vi "Profile Auton - Distance.vi"(8 "error in (no error)":errorcluster, 10 "Time (s)":dbl format="%#_13g", 11 "Distance (ft)":dbl) -> (0 "error out":errorcluster)   [LabVIEW 2017]
uses:
  Robot Global Data.vi
  <vilib>/Rock Robotics/WPI/Utilities/WPI_GetSetVariantRefNum.vi
  <vilib>/Rock Robotics/Network Tables/NT Write Number.vi
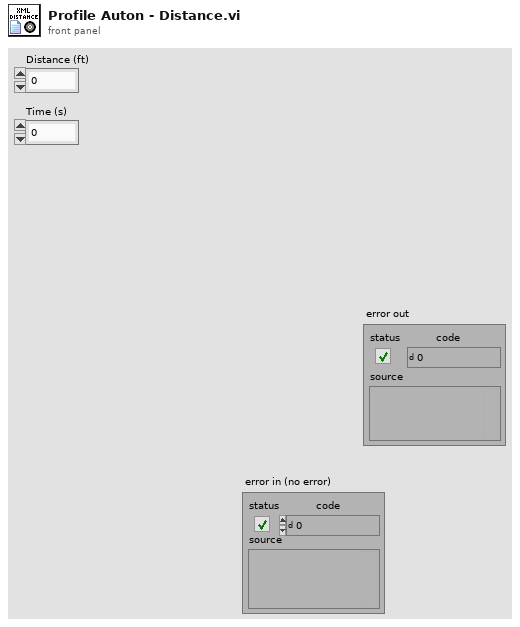
[diagram p1: front panel]
types:
  T1 = typedef "WPI_MotorControlDeviceRef.ctl" = cluster{"DeviceStatus":errorcluster, "Type":T2, "PWM":cluster{"PWM Channel":T3, "DeadBand":T4}, "CAN":cluster{"Device Number":u8, "SetOutput VI Ref":variant, "GetOutput VI Ref":variant, "Enable VI Ref":variant, "Disable VI Ref":variant, "Data":variant}, "Invert":bool, "DIO PWM":cluster{"PWM \"Enable\" Channel":T3, "DIOChannel":T5, "PWM Rate":dbl}}
  T2 = typedef "WPI_MotorControlType.ctl" = enum16{"PWM", "CAN", "DIO PWM"}
  T3 = typedef "FPGA_DIOPWMChannel.ctl" = enum8{"PWM 0", "PWM 1", "PWM 2", "PWM 3", "PWM 4", "PWM 5", "PWM 6", "PWM 7", "PWM 8", "PWM 9", "PWM MXP 0", "PWM MXP 1", "PWM MXP 2", "PWM MXP 3", "PWM MXP 4", "PWM MXP 5", "PWM MXP 6", "PWM MXP 7", "PWM MXP 8", "PWM MXP 9", "Invalid"}
  T4 = typedef "WPI_PWMDeadband.ctl" = cluster{"Name":string, "maxPositivePwm":i32, "minPositivePwm":i32, "centerPwm":i32, "maxNegativePwm":i32, "minNegativePwm":i32, "angularRange":u16}
  T5 = typedef "FPGA_DIOChannel.ctl" = enum8{"DIO 0", "DIO 1", "DIO 2", "DIO 3", "DIO 4", "DIO 5", "DIO 6", "DIO 7", "DIO 8", "DIO 9", "DIO MXP 0", "DIO MXP 1", "DIO MXP 2", "DIO MXP 3", "DIO MXP 4", "DIO MXP 5", "DIO MXP 6", "DIO MXP 7", "DIO MXP 8", "DIO MXP 9", "DIO MXP 10", "DIO MXP 11", "DIO MXP 12", "DIO MXP 13", "DIO MXP 14", "DIO MXP 15", "SPI Port CS1", "SPI Port CS2", "SPI Port CS3", "SPI Port MISO", "SPI Port MOSI", "Invalid"}
  T6 = typedef "WPI_RobotDriveDevRef.ctl" = cluster{"DevStatus":errorcluster, "Motors[]":T1[], "Square Inputs":bool, "Max Output":dbl}
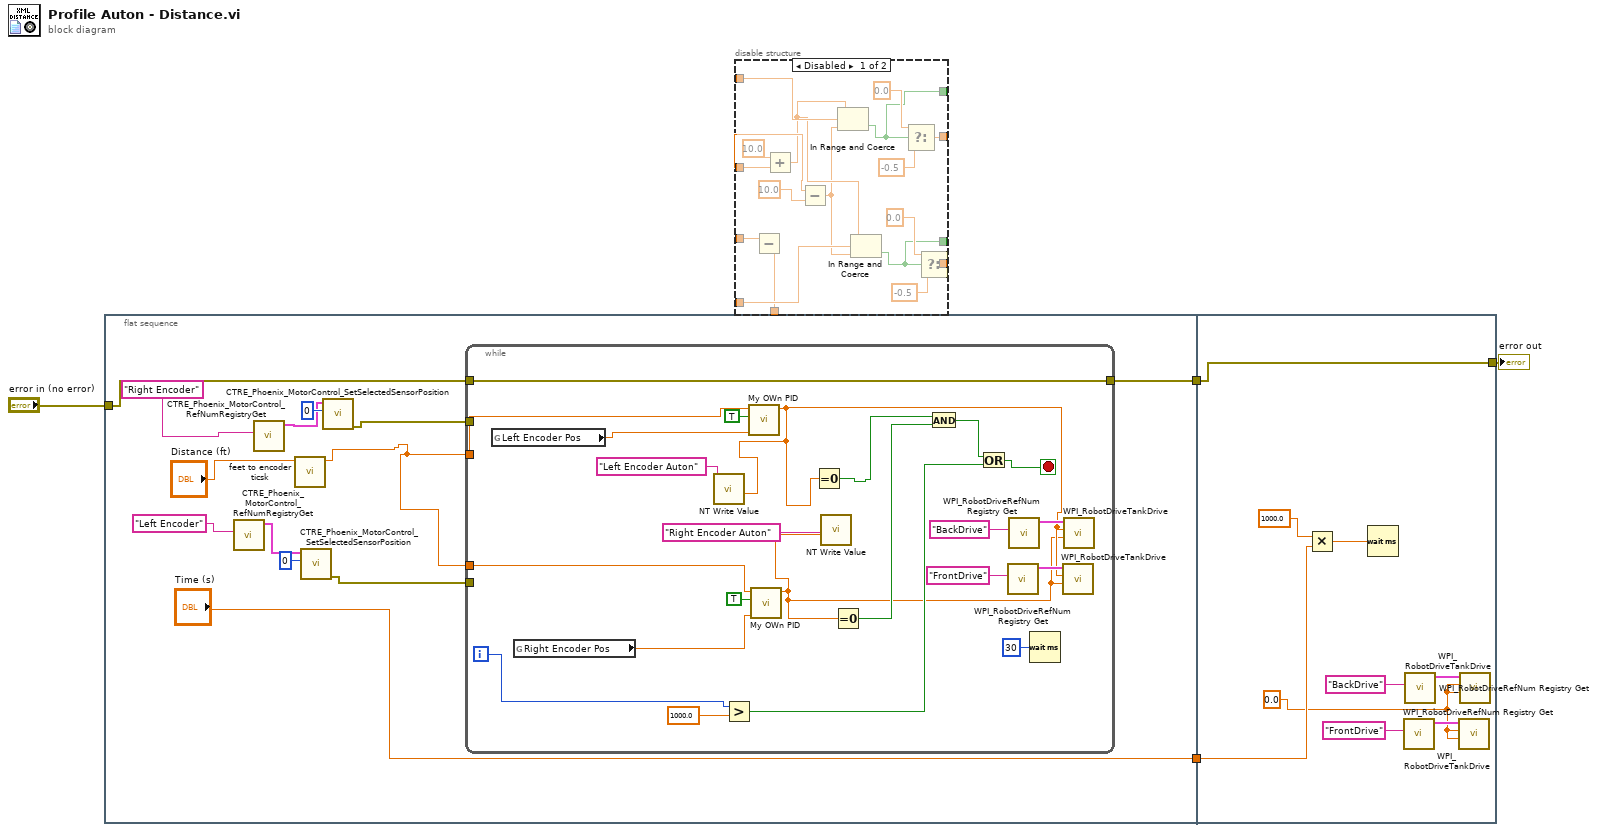
[diagram p0: block diagram]
diagram:
  n1 = flat-sequence {
    tunnel: ["Time (s)"] -> w4
    tunnel: "error in (no error)" -> [w15]
    tunnel: [w14] -> w2
    tunnel: w4 -> [w48]
    tunnel: w2 -> [w46]
    tunnel: [w46] -> w1
    frame #0 {
      n2 = call <vilib>:"CTRE_Phoenix_MotorControl_RefNumRegistryGet.vi"("refnum name"="Left Encoder") -> ("PhoenixMotorControlDevRef"=w6:T1)  [unwired: 9 in, 1 out]
      n3 = call <vilib>:"CTRE_Phoenix_MotorControl_RefNumRegistryGet.vi"("refnum name"="Right Encoder") -> ("PhoenixMotorControlDevRef"=w7:T1)  [unwired: 9 in, 1 out]
      n4 = call "feet to encoder ticsk.vi"("Distance in feet wanted"="Distance (ft)") -> ("Encoder Ticks"=w13:dbl)  [unwired: 10 in]
      n5 = call <vilib>:"CTRE_Phoenix_MotorControl_SetSelectedSensorPosition.vi"("New Sensor Position"=0, "PhoenixMotorControlDevRef"=w6) -> ("error out"=w12:errorcluster)  [unwired: 8 in, 1 out]
      n6 = call <vilib>:"CTRE_Phoenix_MotorControl_SetSelectedSensorPosition.vi"("New Sensor Position"=0, "PhoenixMotorControlDevRef"=w7) -> ("error out"=w9:errorcluster)  [unwired: 8 in, 1 out]
      n7 = while {
        tunnel: w13 -> [w39]
        tunnel: w13 -> [w38]
        tunnel: w15 -> [w37]
        tunnel: [w37] -> w14
        tunnel: w12 -> [_]
        tunnel: w9 -> [_]
        i -> [w27]
        stop <- w24 stop-if-true
        n8 = global read "Robot Global Data.vi" "Left Encoder Pos"() -> (w34:dbl)
        n9 = global read "Robot Global Data.vi" "Right Encoder Pos"() -> (w33:dbl)
        n10 = Greater?(x=w27, y=1000.0) -> (0:w26:bool)
        n11 = call "My OWn PID.vi"("Current Input"=w34, "Encoders (t) gyro (f)"=TRUE, "Wanted End"=w38) -> ("Output"=w19:dbl)  [unwired: 8 in]
        n12 = call-poly <vilib>:"NT Write Value.vi"("Numeric"=w19, "Name"="Left Encoder Auton") -> ()  [unwired: 9 in, 1 out]
        n13 = call "My OWn PID.vi"("Current Input"=w33, "Encoders (t) gyro (f)"=TRUE, "Wanted End"=w39) -> ("Output"=w18:dbl)  [unwired: 8 in]
        n14 = Equal To 0?(x=w19) -> (x = 0?=w30:bool)
        n15 = call-poly <vilib>:"NT Write Value.vi"("Numeric"=w18, "Name"="Right Encoder Auton") -> ()  [unwired: 9 in, 1 out]
        n16 = Equal To 0?(x=w18) -> (x = 0?=w29:bool)
        n17 = And(x=w30, y=w29) -> (x .and. y?=w25:bool)
        n18 = Or(x=w25, y=w26) -> (x .or. y?=w24:bool)
        n19 = call <vilib>:"WPI_RobotDriveRefNum Registry Get.vi"("refnum name"="FrontDrive") -> ("RobotDriveDevRef"=w23:T6)  [unwired: 9 in, 1 out]
        n20 = call <vilib>:"WPI_RobotDriveRefNum Registry Get.vi"("refnum name"="BackDrive") -> ("RobotDriveDevRef"=w22:T6)  [unwired: 9 in, 1 out]
        n21 = Wait (ms)(milliseconds to wait=u32 30) -> ()  [unwired: 1 out]
        n22 = call <vilib>:"WPI_RobotDriveTankDrive.vi"("Right axis value"=w18, "Left axis value"=w19, "RobotDriveDevRef"=w23) -> ()  [unwired: 6 in, 3 out]
        n23 = call <vilib>:"WPI_RobotDriveTankDrive.vi"("Right axis value"=w18, "Left axis value"=w19, "RobotDriveDevRef"=w22) -> ()  [unwired: 6 in, 3 out]
      }
    }
    frame #1 {
      w41 = 0.0
      n24 = Multiply(x=1000.0, y=w48) -> (x*y=w49:dbl)
      n25 = Wait (ms)(milliseconds to wait=w49) -> ()  [unwired: 1 out]
      n26 = call <vilib>:"WPI_RobotDriveRefNum Registry Get.vi"("refnum name"="FrontDrive") -> ("RobotDriveDevRef"=w42:T6)  [unwired: 9 in, 1 out]
      n27 = call <vilib>:"WPI_RobotDriveRefNum Registry Get.vi"("refnum name"="BackDrive") -> ("RobotDriveDevRef"=w43:T6)  [unwired: 9 in, 1 out]
      n28 = call <vilib>:"WPI_RobotDriveTankDrive.vi"("Right axis value"=w41, "Left axis value"=w41, "RobotDriveDevRef"=w42) -> ()  [unwired: 6 in, 3 out]
      n29 = call <vilib>:"WPI_RobotDriveTankDrive.vi"("Right axis value"=w41, "Left axis value"=w41, "RobotDriveDevRef"=w43) -> ()  [unwired: 6 in, 3 out]
    }
  }
  n30 = disable-structure shown="Disabled" {
    disable-tunnel: _ -> [w64 _]
    disable-tunnel: _ -> [w62 _]
    disable-tunnel: _ -> [w58 _]
    disable-tunnel: [w55 _] -> _
    disable-tunnel: [w54 _] -> _
    disable-tunnel: [w53 _] -> _
    disable-tunnel: [w52 _] -> _
    disable-tunnel: _ -> [w51 _]
    disable-tunnel: [w50 _] -> _
    frame Disabled {
      n31 = Subtract(x=w51) -> (x-y=w50:dbl)  [unwired: 1 in]
      n32 = Add(x=10.0, y=w62) -> (x+y=w57:dbl)
      n33 = Subtract(x=w62, y=10.0) -> (x-y=w56:dbl)
      n34 = In Range and Coerce(upper limit=w57, x=w64, lower limit=w56) -> (In Range?=w55:bool)  [unwired: 1 out]
      n35 = In Range and Coerce(upper limit=w57, x=w58, lower limit=w56) -> (In Range?=w54:bool)  [unwired: 1 out]
      n36 = Select(t=0.0, s=w55, f=-0.5) -> (s? t:f=w53:dbl)
      n37 = Select(t=0.0, s=w54, f=-0.5) -> (s? t:f=w52:dbl)
    }
    frame Enabled {
    }
  }
  "error out" <- w1
